vi "Offset Locking Frequency Adjustment.vi"() -> ()   [LabVIEW 2012]
doc: "This application VI for the Hewlett Packard ESG/ESG-D Series Signal Generator will open a VISA session and configure the signal generator to output a FM signal with the following characteristics:\nCarrier frequency set to 104.9 MHz\nPower level set to 0 dBm\nFM deviation set to 75 kHz\nFM rate set to 10 kHz\n\nIt will then check for errors and close the session.\n\nNotes:\nThe VI is available for ESG-A and ESG-D Series instruments only because of Config Frequency.vi."
uses:
  Agilent ESG Series.lvlib
panel:
  in  "Stop":bool
  in  "Output Enable":bool=TRUE
  in  "VISA session":refnum<visa-resource-name>
  in  "Amplitude (dBm)":dbl=7.0 format="%.2f"
  in  "Frequency (MHz)":dbl=224.0 format="%.11f"
  in  "error in (no error)":errorcluster {"code" format="%.0x"}
  out "error out":errorcluster {"code" format="%.0x"}
  # "(c) 2005 - 2013 National Instruments.  ALL RIGHTS RESERVED."
  # "Series Signal Generator"
  # "ESG/ESG-D"
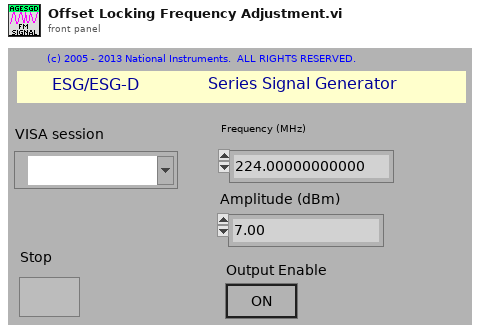
[diagram p1: front panel]
types:
  T1 = enum16{"dBm", "dBuV", "dBuVemf", "mV", "uV", "mVemf", "uVemf"}
  T2 = enum16{"SINE", "TRIANGLE", "SQUARE", "RAMP", "NOISE", "DUAL SINE", "SWEPT SINE"}
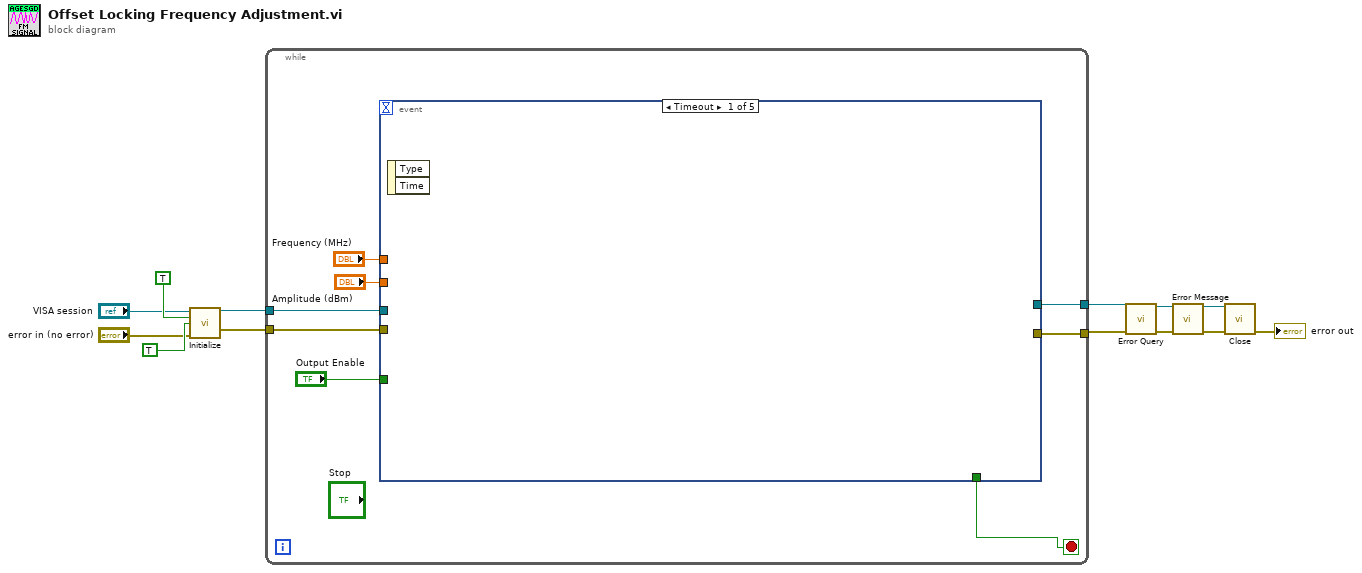
[diagram p0: block diagram]
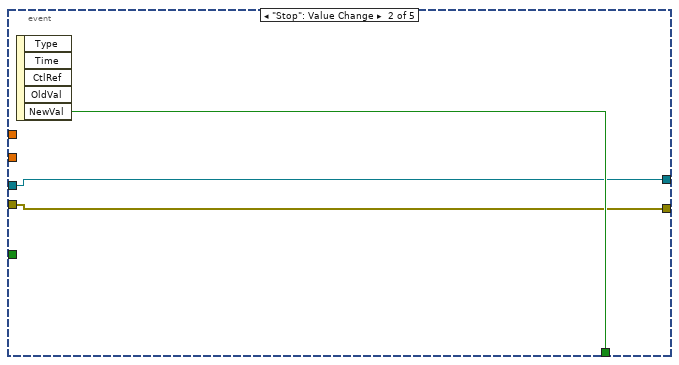
[diagram p2: hidden frame]
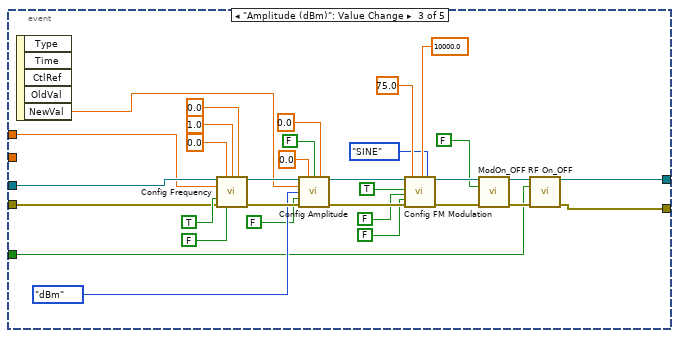
[diagram p3: hidden frame]
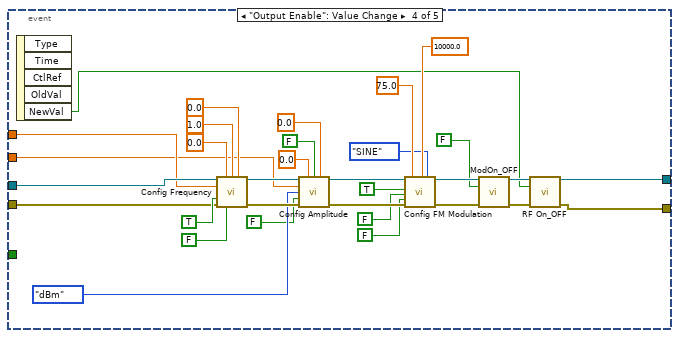
[diagram p4: hidden frame]
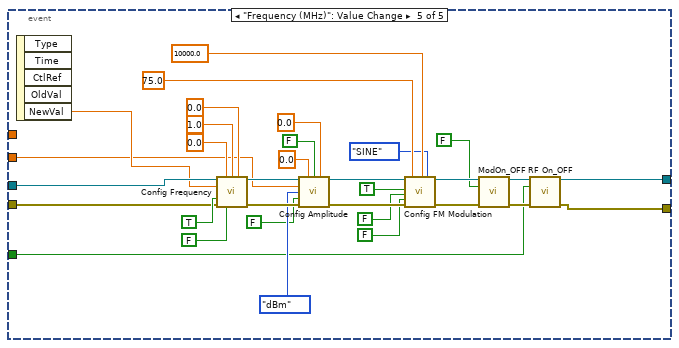
[diagram p5: hidden frame]
diagram:
  n1 = call "Initialize.vi"("VISA Resource Name"="VISA session", "ID Query? (T: Yes)"=TRUE, "Reset? (T: Yes)"=TRUE, "error in (no error)"="error in (no error)") -> ("VISA Resource Name Out"=w3:refnum<visa-resource-name>, "error out"=w2:errorcluster)  [unwired: 10 in]
  n2 = while {
    tunnel: [w21] -> w8
    tunnel: w3 -> [w20]
    tunnel: w2 -> [w19]
    tunnel: [w18] -> w1
    stop <- w16 stop-if-true
    n3 = event shown="[0] Timeout" {
      selector: _ -> [_ _ _ _ _]
      dyn-events: _ -> [_ _ _ _ _]
      timeout: _ -> [_ _ _ _ _]
      tunnel: [_ w22 w31 w63 w95] -> w21
      tunnel: w20 -> [_ w23 w30 w62 w94]
      tunnel: w19 -> [_ w22 w29 w61 w93]
      tunnel: "Output Enable" -> [_ _ w28 _ w90]
      tunnel: [_ w23 w27 w60 w89] -> w18
      tunnel: "Frequency (MHz)" -> [_ _ w25 w59 _]
      tunnel: [_ w24 _ _ _] -> w16
      tunnel: "Amplitude (dBm)" -> [_ _ _ w58 w91]
      event Timeout {
        n4 = event-data() -> ()  [unwired: 1 in, 2 out]
      }
      event "Stop": Value Change {
        n5 = event-data() -> ("NewVal"=w24:bool)  [unwired: 1 in, 4 out]
      }
      event "Amplitude (dBm)": Value Change {
        n6 = event-data() -> ("NewVal"=w26:dbl)  [unwired: 1 in, 4 out]
        n7 = call "Config Frequency.vi"("VISA Resource Name"=w30, "Freq Offset (0.0)"=0.0, "Freq Multiplier (1.0)"=1.0, "Adjust Phase (0.0)"=0.0, "Frequency (1000.0)"=w25, "Freq Ref (T:ON)"=TRUE, "error in (no error)"=w29, "OptPhNoise (F:MD2 > 10khzOffset)"=FALSE) -> ("VISA Resource Name Out"=w56:refnum<visa-resource-name>, "error out"=w55:errorcluster)  [unwired: 6 in]
        n8 = call "Config Amplitude.vi"("VISA Resource Name"=w56, "Ampl Ref Set (0.00)"=0.0, "Ampl Ref (F:OFF)"=FALSE, "Ampl Offset (0.00)"=0.0, "Amplitude (-135.00)"=w26, "Unit (0:dBm)"=T1."dBm", "Atten Hold (F:OFF)"=FALSE, "error in (no error)"=w55) -> ("VISA Resource Name Out"=w54:refnum<visa-resource-name>, "error out"=w53:errorcluster)  [unwired: 6 in]
        n9 = call "Config FM Modulation.vi"("VISA Resource Name"=w54, "Status (T:ON)"=TRUE, "EXT Source Coupling (F:DC)"=FALSE, "FM Deviation Couple (F:OFF)"=FALSE, "error in (no error)"=w53, "FM Deviation (1.0)"=75.0 ("FM Deviation (75)"), "FM Rate (400.0)"=10000.0 ("FM Rate (10000)"), "FM Waveform (0:SINE)"=T2."SINE") -> ("VISA Resource Name Out"=w52:refnum<visa-resource-name>, "error out"=w51:errorcluster)  [unwired: 10 in]
        n10 = call "ModOn_OFF.vi"("VISA Resource Name"=w52, "Status (T:ON)"=FALSE, "error in (no error)"=w51) -> ("VISA Resource Name Out"=w50:refnum<visa-resource-name>, "error out"=w49:errorcluster)  [unwired: 11 in]
        n11 = call "RF On_OFF.vi"("VISA Resource Name"=w50, "Status (T:ON)"=w28, "error in (no error)"=w49) -> ("VISA Resource Name Out"=w27:refnum<visa-resource-name>, "error out"=w31:errorcluster)  [unwired: 11 in]
      }
      event "Output Enable": Value Change {
        n12 = event-data() -> ("NewVal"=w57:bool)  [unwired: 1 in, 4 out]
        n13 = call "Config Frequency.vi"("VISA Resource Name"=w62, "Freq Offset (0.0)"=0.0, "Freq Multiplier (1.0)"=1.0, "Adjust Phase (0.0)"=0.0, "Frequency (1000.0)"=w59, "Freq Ref (T:ON)"=TRUE, "error in (no error)"=w61, "OptPhNoise (F:MD2 > 10khzOffset)"=FALSE) -> ("VISA Resource Name Out"=w88:refnum<visa-resource-name>, "error out"=w87:errorcluster)  [unwired: 6 in]
        n14 = call "Config Amplitude.vi"("VISA Resource Name"=w88, "Ampl Ref Set (0.00)"=0.0, "Ampl Ref (F:OFF)"=FALSE, "Ampl Offset (0.00)"=0.0, "Amplitude (-135.00)"=w58, "Unit (0:dBm)"=T1."dBm", "Atten Hold (F:OFF)"=FALSE, "error in (no error)"=w87) -> ("VISA Resource Name Out"=w86:refnum<visa-resource-name>, "error out"=w85:errorcluster)  [unwired: 6 in]
        n15 = call "Config FM Modulation.vi"("VISA Resource Name"=w86, "Status (T:ON)"=TRUE, "EXT Source Coupling (F:DC)"=FALSE, "FM Deviation Couple (F:OFF)"=FALSE, "error in (no error)"=w85, "FM Deviation (1.0)"=75.0 ("FM Deviation (75)"), "FM Rate (400.0)"=10000.0 ("FM Rate (10000)"), "FM Waveform (0:SINE)"=T2."SINE") -> ("VISA Resource Name Out"=w84:refnum<visa-resource-name>, "error out"=w83:errorcluster)  [unwired: 10 in]
        n16 = call "ModOn_OFF.vi"("VISA Resource Name"=w84, "Status (T:ON)"=FALSE, "error in (no error)"=w83) -> ("VISA Resource Name Out"=w82:refnum<visa-resource-name>, "error out"=w81:errorcluster)  [unwired: 11 in]
        n17 = call "RF On_OFF.vi"("VISA Resource Name"=w82, "Status (T:ON)"=w57, "error in (no error)"=w81) -> ("VISA Resource Name Out"=w60:refnum<visa-resource-name>, "error out"=w63:errorcluster)  [unwired: 11 in]
      }
      event "Frequency (MHz)": Value Change {
        n18 = event-data() -> ("NewVal"=w92:dbl)  [unwired: 1 in, 4 out]
        n19 = call "Config Frequency.vi"("VISA Resource Name"=w94, "Freq Offset (0.0)"=0.0, "Freq Multiplier (1.0)"=1.0, "Adjust Phase (0.0)"=0.0, "Frequency (1000.0)"=w92, "Freq Ref (T:ON)"=TRUE, "error in (no error)"=w93, "OptPhNoise (F:MD2 > 10khzOffset)"=FALSE) -> ("VISA Resource Name Out"=w120:refnum<visa-resource-name>, "error out"=w119:errorcluster)  [unwired: 6 in]
        n20 = call "Config Amplitude.vi"("VISA Resource Name"=w120, "Ampl Ref Set (0.00)"=0.0, "Ampl Ref (F:OFF)"=FALSE, "Ampl Offset (0.00)"=0.0, "Amplitude (-135.00)"=w91, "Unit (0:dBm)"=T1."dBm", "Atten Hold (F:OFF)"=FALSE, "error in (no error)"=w119) -> ("VISA Resource Name Out"=w118:refnum<visa-resource-name>, "error out"=w117:errorcluster)  [unwired: 6 in]
        n21 = call "Config FM Modulation.vi"("VISA Resource Name"=w118, "Status (T:ON)"=TRUE, "EXT Source Coupling (F:DC)"=FALSE, "FM Deviation Couple (F:OFF)"=FALSE, "error in (no error)"=w117, "FM Deviation (1.0)"=75.0 ("FM Deviation (75)"), "FM Rate (400.0)"=10000.0 ("FM Rate (10000)"), "FM Waveform (0:SINE)"=T2."SINE") -> ("VISA Resource Name Out"=w116:refnum<visa-resource-name>, "error out"=w115:errorcluster)  [unwired: 10 in]
        n22 = call "ModOn_OFF.vi"("VISA Resource Name"=w116, "Status (T:ON)"=FALSE, "error in (no error)"=w115) -> ("VISA Resource Name Out"=w114:refnum<visa-resource-name>, "error out"=w113:errorcluster)  [unwired: 11 in]
        n23 = call "RF On_OFF.vi"("VISA Resource Name"=w114, "Status (T:ON)"=w90, "error in (no error)"=w113) -> ("VISA Resource Name Out"=w89:refnum<visa-resource-name>, "error out"=w95:errorcluster)  [unwired: 11 in]
      }
    }
  }
  n24 = call "Error Query.vi"("VISA Resource Name"=w1, "error in (no error)"=w8) -> ("VISA Resource Name Out"=w10:refnum<visa-resource-name>, "error out"=w13:errorcluster)  [unwired: 10 in, 2 out]
  n25 = call "Error Message.vi"("VISA Resource Name"=w10, "error in (no error)"=w13) -> ("VISA Resource Name Out"=w11:refnum<visa-resource-name>, "error out"=w12:errorcluster)  [unwired: 9 in, 3 out]
  n26 = call "Close.vi"("VISA Resource Name"=w11, "error in (no error)"=w12) -> ("error out"=→"error out":errorcluster)  [unwired: 13 in]
